vi "Close Hardware.vi"(8 "error in (no error)":errorcluster, 11 "Instrument.FrameworkTemplate":refnum<class "Temperhum.Thorlabs.lvclass">) -> (0 "error out":errorcluster, 3 "Instrument.FrameworkTemplate out":refnum<class "Temperhum.Thorlabs.lvclass">)   [LabVIEW 2019, in "Temperhum.Thorlabs.lvclass"]
uses:
  Temperhum.Thorlabs.lvclass
  Temperhum.Thorlabs.lvclass/Temperhum.Thorlabs.ctl
  Instrument.Temperhum/Instrument.Temperhum.lvclass
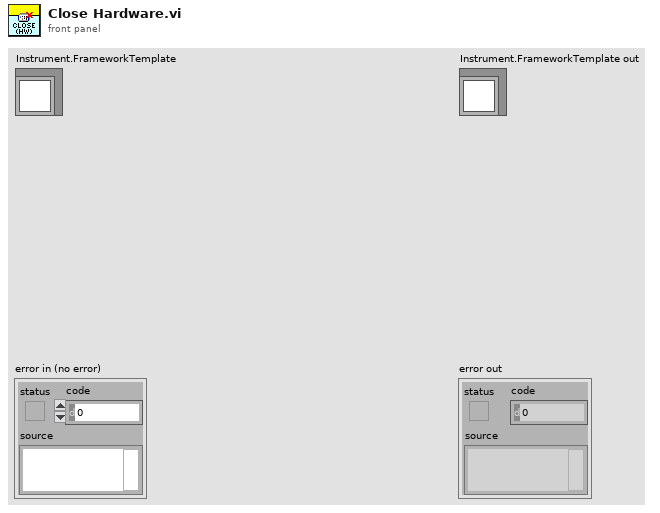
[diagram p1: front panel]
types:
  T1 = typedef "Temperhum.Thorlabs.lvclass/Thorlabs Type --enum.ctl" = enum16{"A", "B"}
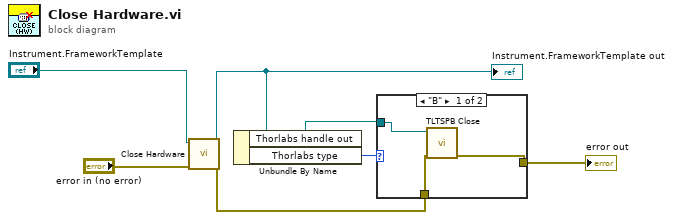
[diagram p0: block diagram]
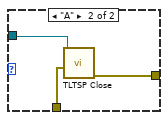
[diagram p2: hidden frame]
diagram:
  n1 = call-parent "Close Hardware.vi"("error in (no error)"="error in (no error)", "Instrument.FrameworkTemplate"="Instrument.FrameworkTemplate") -> ("error out"=w3:errorcluster, "Instrument.FrameworkTemplate out"=w5:refnum<class "Temperhum.Thorlabs.lvclass">)  [unwired: 8 in]
  "Instrument.FrameworkTemplate out" <- w5
  n2 = Unbundle By Name(w5) -> ("Thorlabs handle out"=w4:refnum<visa-resource-name>, "Thorlabs type"=w1:T1)
  n3 = case shown="\"B\"" w1 {
    tunnel: w4 -> [w10 w13]
    tunnel: w3 -> [w9 w12]
    tunnel: [w8 w11] -> w2
    frame "B" {
      n4 = call "TLTSPB Close.vi"("error in (no error)"=w9, "instrument handle"=w10) -> ("error out"=w8:errorcluster)  [unwired: 9 in]
    }
    frame "A" {
      n5 = call "TLTSP Close.vi"("error in (no error)"=w12, "instrument handle"=w13) -> ("error out"=w11:errorcluster)  [unwired: 9 in]
    }
  }
  "error out" <- w2
